vi "Read Properties.vi"(8 "error in":errorcluster, 11 "Item in":refnum<class "Item.lvclass">) -> (0 "error out":errorcluster, 2 "Properties":refnum<class "Property.lvclass">[](array[class]), 3 "Item out":refnum<class "Item.lvclass">)   [LabVIEW 2024, in "Parser.lvlib" / "Item.lvclass"]
uses:
  Item.lvclass
  Property/Property.lvclass
  Item.lvclass/Item.ctl
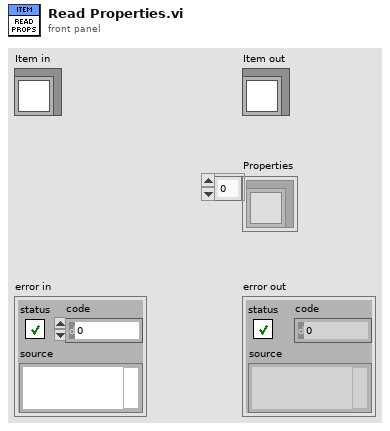
[diagram p1: front panel]
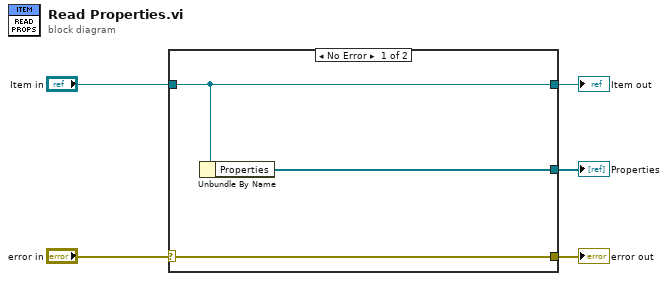
[diagram p0: block diagram]
diagram:
  n1 = case shown="No Error" "error in" {
    selector: "error in" -> [w8 w10]
    tunnel: [w8 w10] -> w4
    tunnel: [w7 w9] -> w2
    tunnel: "Item in" -> [w7 w9]
    tunnel: [w6 _] -> w1
    frame No Error {
      n2 = Unbundle By Name(w7) -> ("Properties"=w6:refnum<class "Property.lvclass">[])
    }
    frame Error {
    }
  }
  "error out" <- w4
  "Item out" <- w2
  "Properties" <- w1
